vi "Target.vi"() -> ()   [LabVIEW 2025]
uses:
  <vilib>/Platform/TimedLoop/XDataNode/timing_clust.ctl
  <vilib>/Platform/TimedLoop/XDataNode/nitl_modes.ctl
  <vilib>/Platform/TimedLoop/XDataNode/wakeup.ctl
  <vilib>/rvi/Emulation/niFpgaSctlEmulationGetInTimedLoop.vi
  <vilib>/rvi/Emulation/niFpgaEmulationReportErrorSimple.vi
  <vilib>/rvi/Emulation/niFpgaGetClockAttributes.vi
  <vilib>/rvi/Emulation/niFpgaCriticalErrorInLSC.vi
  <vilib>/rvi/linearAlgebra/MatrixMultiply/simVIs/SubVI/nifxpla_MatrixMultiply_SimMatrixSizes.vi
  <vilib>/rvi/linearAlgebra/MatrixMultiply/simVIs/SubVI/nifxpla_MatrixMultiply_Sim4WireAdapterVector.vi
  <vilib>/rvi/linearAlgebra/MatrixMultiply/simVIs/SubVI/nifxpla_MatrixMultiply_SimFrameHandShake.vi
  <vilib>/rvi/linearAlgebra/MatrixMultiply/simVIs/SubVI/nifxpla_MatrixMultiply_SimEndlessCounter.vi
  <vilib>/rvi/linearAlgebra/MatrixMultiply/simVIs/SubVI/nifxpla_MatrixMultiply_SimVectorDataBuffer.vi
  <vilib>/rvi/ClientSDK/Core/DevComputerLib/Private/Multiply(dfxp64).vi
  <vilib>/rvi/ClientSDK/Core/DevComputerLib/Private/Dfxp128ToDfxp256.vi
  <vilib>/rvi/ClientSDK/Core/DevComputerLib/Private/Add(dfxp256).vi
  <vilib>/rvi/ClientSDK/Core/DevComputerLib/Private/Subtract(dfxp256).vi
  <vilib>/rvi/ClientSDK/Core/DevComputerLib/Private/ToDfxp64(dfxp256).vi
  <vilib>/platform/TimedLoop/XDataNode/XDataNode.xnode
  <vilib>/rvi/linearAlgebra/MatrixMultiply/XNode/nifxpla_MatrixMultiply.xnode
  <vilib>/rvi/linearAlgebra/MatrixMultiply/simVIs/nifxpla_MatrixMultiply_SimTemplateEinEout.vi
  <vilib>/rvi/linearAlgebra/MatrixMultiply/simVIs/nifxpla_MatrixMultiply_SimTemplateEinVout.vi
  <vilib>/rvi/linearAlgebra/MatrixMultiply/simVIs/nifxpla_MatrixMultiply_SimTemplateVinEout.vi
  <vilib>/rvi/linearAlgebra/MatrixMultiply/simVIs/nifxpla_MatrixMultiply_SimTemplateVinVout.vi
  <vilib>/Platform/TimedLoop/XDataNode/XDNodeRunTimeDep.lvlib
panel:
  out "C":fxp<+/-,32,16>[](array[numeric])
  out "Cycle Count":i32
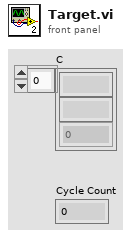
[diagram p1: front panel]
types:
  T1 = typedef "XDNodeRunTimeDep.lvlib/timing_clust.ctl" = cluster{"Expected End [f-1]":u64, "Actual End [f-1]":u64, "Finished Late? [f-1]":bool, "Expected End [i-1]":u64, "Actual End [i-1]":u64, "Finished Late? [i-1]":bool, "Expected Start [i]":u64, "Actual Start [i]":u64, "Expected Start [f]":u64, "Actual Start [f]":u64, "Source Name":string, "Structure Name":string, "Period":i64, "Deadline":i64, "Offset":i64, "Start":i64, "Priority":i32, "Timeout":i32, "Mode":T2, "Wakeup Reason":T3, "Error":errorcluster, "Source Type":string, "Secondary Source Type":string, "Global End Time":u64, "Global Start Time":u64, "Frame Duration":u64, "Iteration Duration":u64, "Assigned CPU":i32, "I/O Scan Engine Mode":u32}
  T2 = typedef "XDNodeRunTimeDep.lvlib/nitl_modes.ctl" = enum32{"No Change", "Process missed periods, maintain original phase", "Discard missed periods, maintain original phase", "Process missed periods, ignore original phase", "Discard missed periods, ignore original phase"}
  T3 = typedef "XDNodeRunTimeDep.lvlib/wakeup.ctl" = enum32{"Normal", "Aborted", "Asynchronous wakeup", "Timing source error", "Timed loop error", "Timeout"}
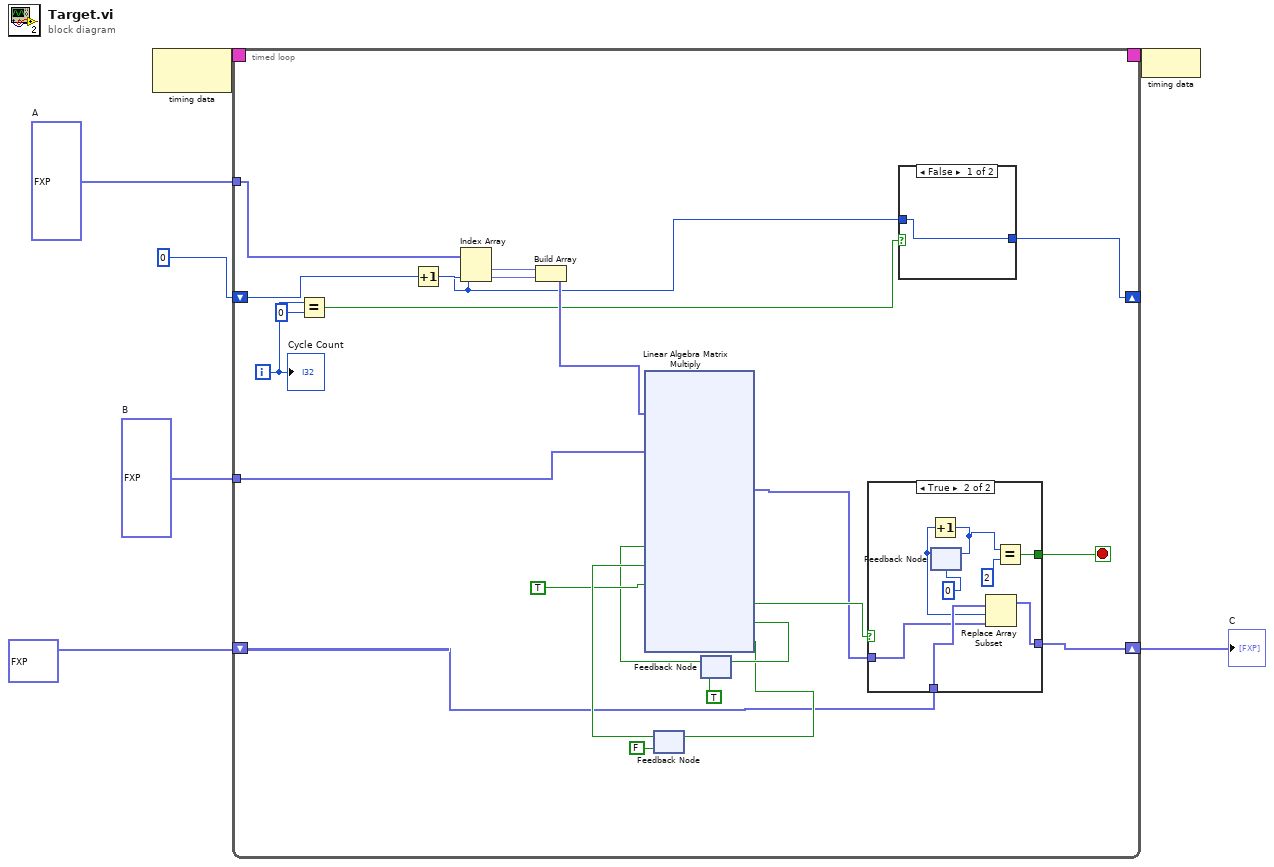
[diagram p0: block diagram]
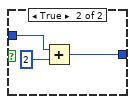
[diagram p2: hidden frame]
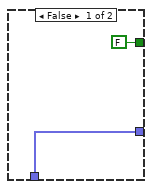
[diagram p3: hidden frame]
diagram:
  w3 = fxp<+/-,32,16>[] [1.0, 2.0, 3.0, 4.0]  # A
  w4 = fxp<+/-,32,16>[] [1.0, 2.0]  # B
  n1 = node-c288() -> (w7:T1)  [unwired: 1 in]
  n2 = timed-loop {
    timing: w7 -> [_]
    timing-out: [_] -> w6
    shift-right: [w22] -> w2
    shift-left: fxp<+/-,32,16>[] [0.0, 0.0] -> [w21]
    tunnel: w4 -> [w19]
    tunnel: w3 -> [w15]
    shift-right: [w9] -> _
    shift-left: 0 ("length") -> [w10]
    i -> [w17]
    stop <- w20 stop-if-true
    n3 = Equal?(x=w17, y=0) -> (x = y?=w8:bool)
    n4 = Increment(x=w10) -> (x+1=w11:i32)
    n5 = Index Array "Index Array"(array=w15, index #1=w10, index #2=w11) -> (element #1=w14:fxp<+/-,32,16>, element #2=w13:fxp<+/-,32,16>)
    n6 = Build Array(w14, w13) -> (w12:fxp<+/-,32,16>[])
    n7 = feedback #1(FALSE ("ready for b")) -> (w28:bool)
    n8 = feedback #2(TRUE ("ready for a")) -> (w18:bool)
    n9 = xnode ("Linear Algebra Matrix Multiply")("ar"=w12, "br"=w19, "a valid"=w18, "b valid"=w28, "ready for output (T)"=TRUE) -> ("cr"=w23:fxp<+/-,32,16>[], "output valid"=w24:bool, "ready for a"=w30:bool, "ready for b"=w29:bool)  [unwired: 2 in, 2 out]
    n10 = feedback-in #1(w29) -> ()
    n11 = feedback-in #2(w30) -> ()
    n12 = case shown="True" w24 {
      tunnel: w23 -> [_ w39]
      tunnel: [w36 w43] -> w22
      tunnel: w21 -> [w36 w44]
      tunnel: [FALSE w40] -> w20
      frame False {
      }
      frame True {
        n13 = feedback #3(0 ("x")) -> (w38:i32)
        n14 = Increment(x=w38) -> (x+1=w37:i32)
        n15 = feedback-in #3(w37) -> ()
        n16 = Replace Array Subset(array=w44, new element=w39, index=w38) -> (w43:fxp<+/-,32,16>[])
        n17 = Equal?(x=w37, y=2) -> (x = y?=w40:bool)
      }
    }
    n18 = case shown="False" w8 {
      tunnel: w10 -> [w31 w34]
      tunnel: [w31 w33] -> w9
      frame False {
      }
      frame True {
        n19 = Add(x=w34, y=2) -> (x+y=w33:i32)
      }
    }
    "Cycle Count" <- w17
  }
  "C" <- w2
  n20 = node-c288(w6) -> ()
